vi "LinearQuadraticRegulator_New_N.vi"(4 "dt_Seconds":dbl=0.02, 5 "States":i32, 6 "N":T1, 7 "Inputs":i32, 8 "R":T1, 9 "Q":T1, 10 "B":T1, 11 "A":T1) -> (0 "Error":errorcluster, 3 "LinearQuadraticRegulator":T2)   [LabVIEW 2019, in "Trajectory_Library.lvlib"]
doc: "Contains the controller coefficients and logic for a linear-quadratic regulator (LQR). LQRs use the control law u = K(r - x).\n \nFor more on the underlying math, read https://file.tavsys.net/control/controls-engineering-in-frc.pdf.\n\nConstructs a controller with the given coefficients and plant.\n\nInputs:\n - A -- Continuous system matrix of the plant being controlled.\n - B -- Continuous input matrix of the plant being controlled.\n - Q -- The state cost matrix.\n - R -- The input cost matrix.\n - N -- The state-input cross-term cost matrix.\n - dtSeconds -- Discretization timestep.\n\nOutputs:\n - LinearQuadraticRegulator -- controller data cluster\n - Error -- if TRUE, and error occured"
uses:
  Trajectory_Library.lvlib
  <vilib>/Analysis/Matrix/Datatypes/RealMatrix.ctl
  <vilib>/Analysis/Matrix/NI_Matrix.lvlib
  TypeDef/LINEAR_QUADRATIC_REGULATOR.ctl
  <vilib>/Analysis/NI_AALPro.lvlib
  <vilib>/Analysis/NI_AALBase.lvlib
  <vilib>/Analysis/baseanly.llb/Real A x B.vi
  <vilib>/Analysis/Matrix/Numeric/Add/Add - RM,RM.vi
  <vilib>/Analysis/7linalg.llb/Real Transpose Matrix.vi
  <vilib>/Analysis/7linalg.llb/Solve Linear Equations (multiple right hand).vi
panel:
  # "<States,States>"
  # "<States,Inputs>"
  # "<States,Inputs>"
  # "<States,States>"
  # "<Inputs,Inputs>"
  # "Ref State <States,1>"
  # "Comp and capped \noutput <Inputs,1>"
  # "Controller gain\n<Inputs,States>"
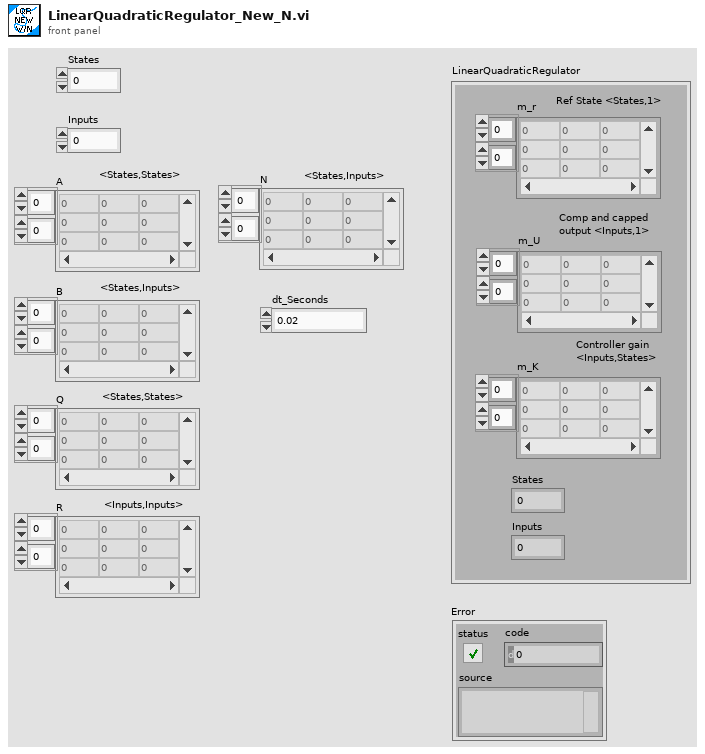
[diagram p1: front panel]
types:
  T1 = typedef "NI_Matrix.lvlib/RealMatrix.ctl" = dbl[][]
  T2 = typedef "Trajectory_Library.lvlib/LINEAR_QUADRATIC_REGULATOR.ctl" = cluster{"m_r":T1, "m_U":T1, "m_K":T1, "States":i32, "Inputs":i32}
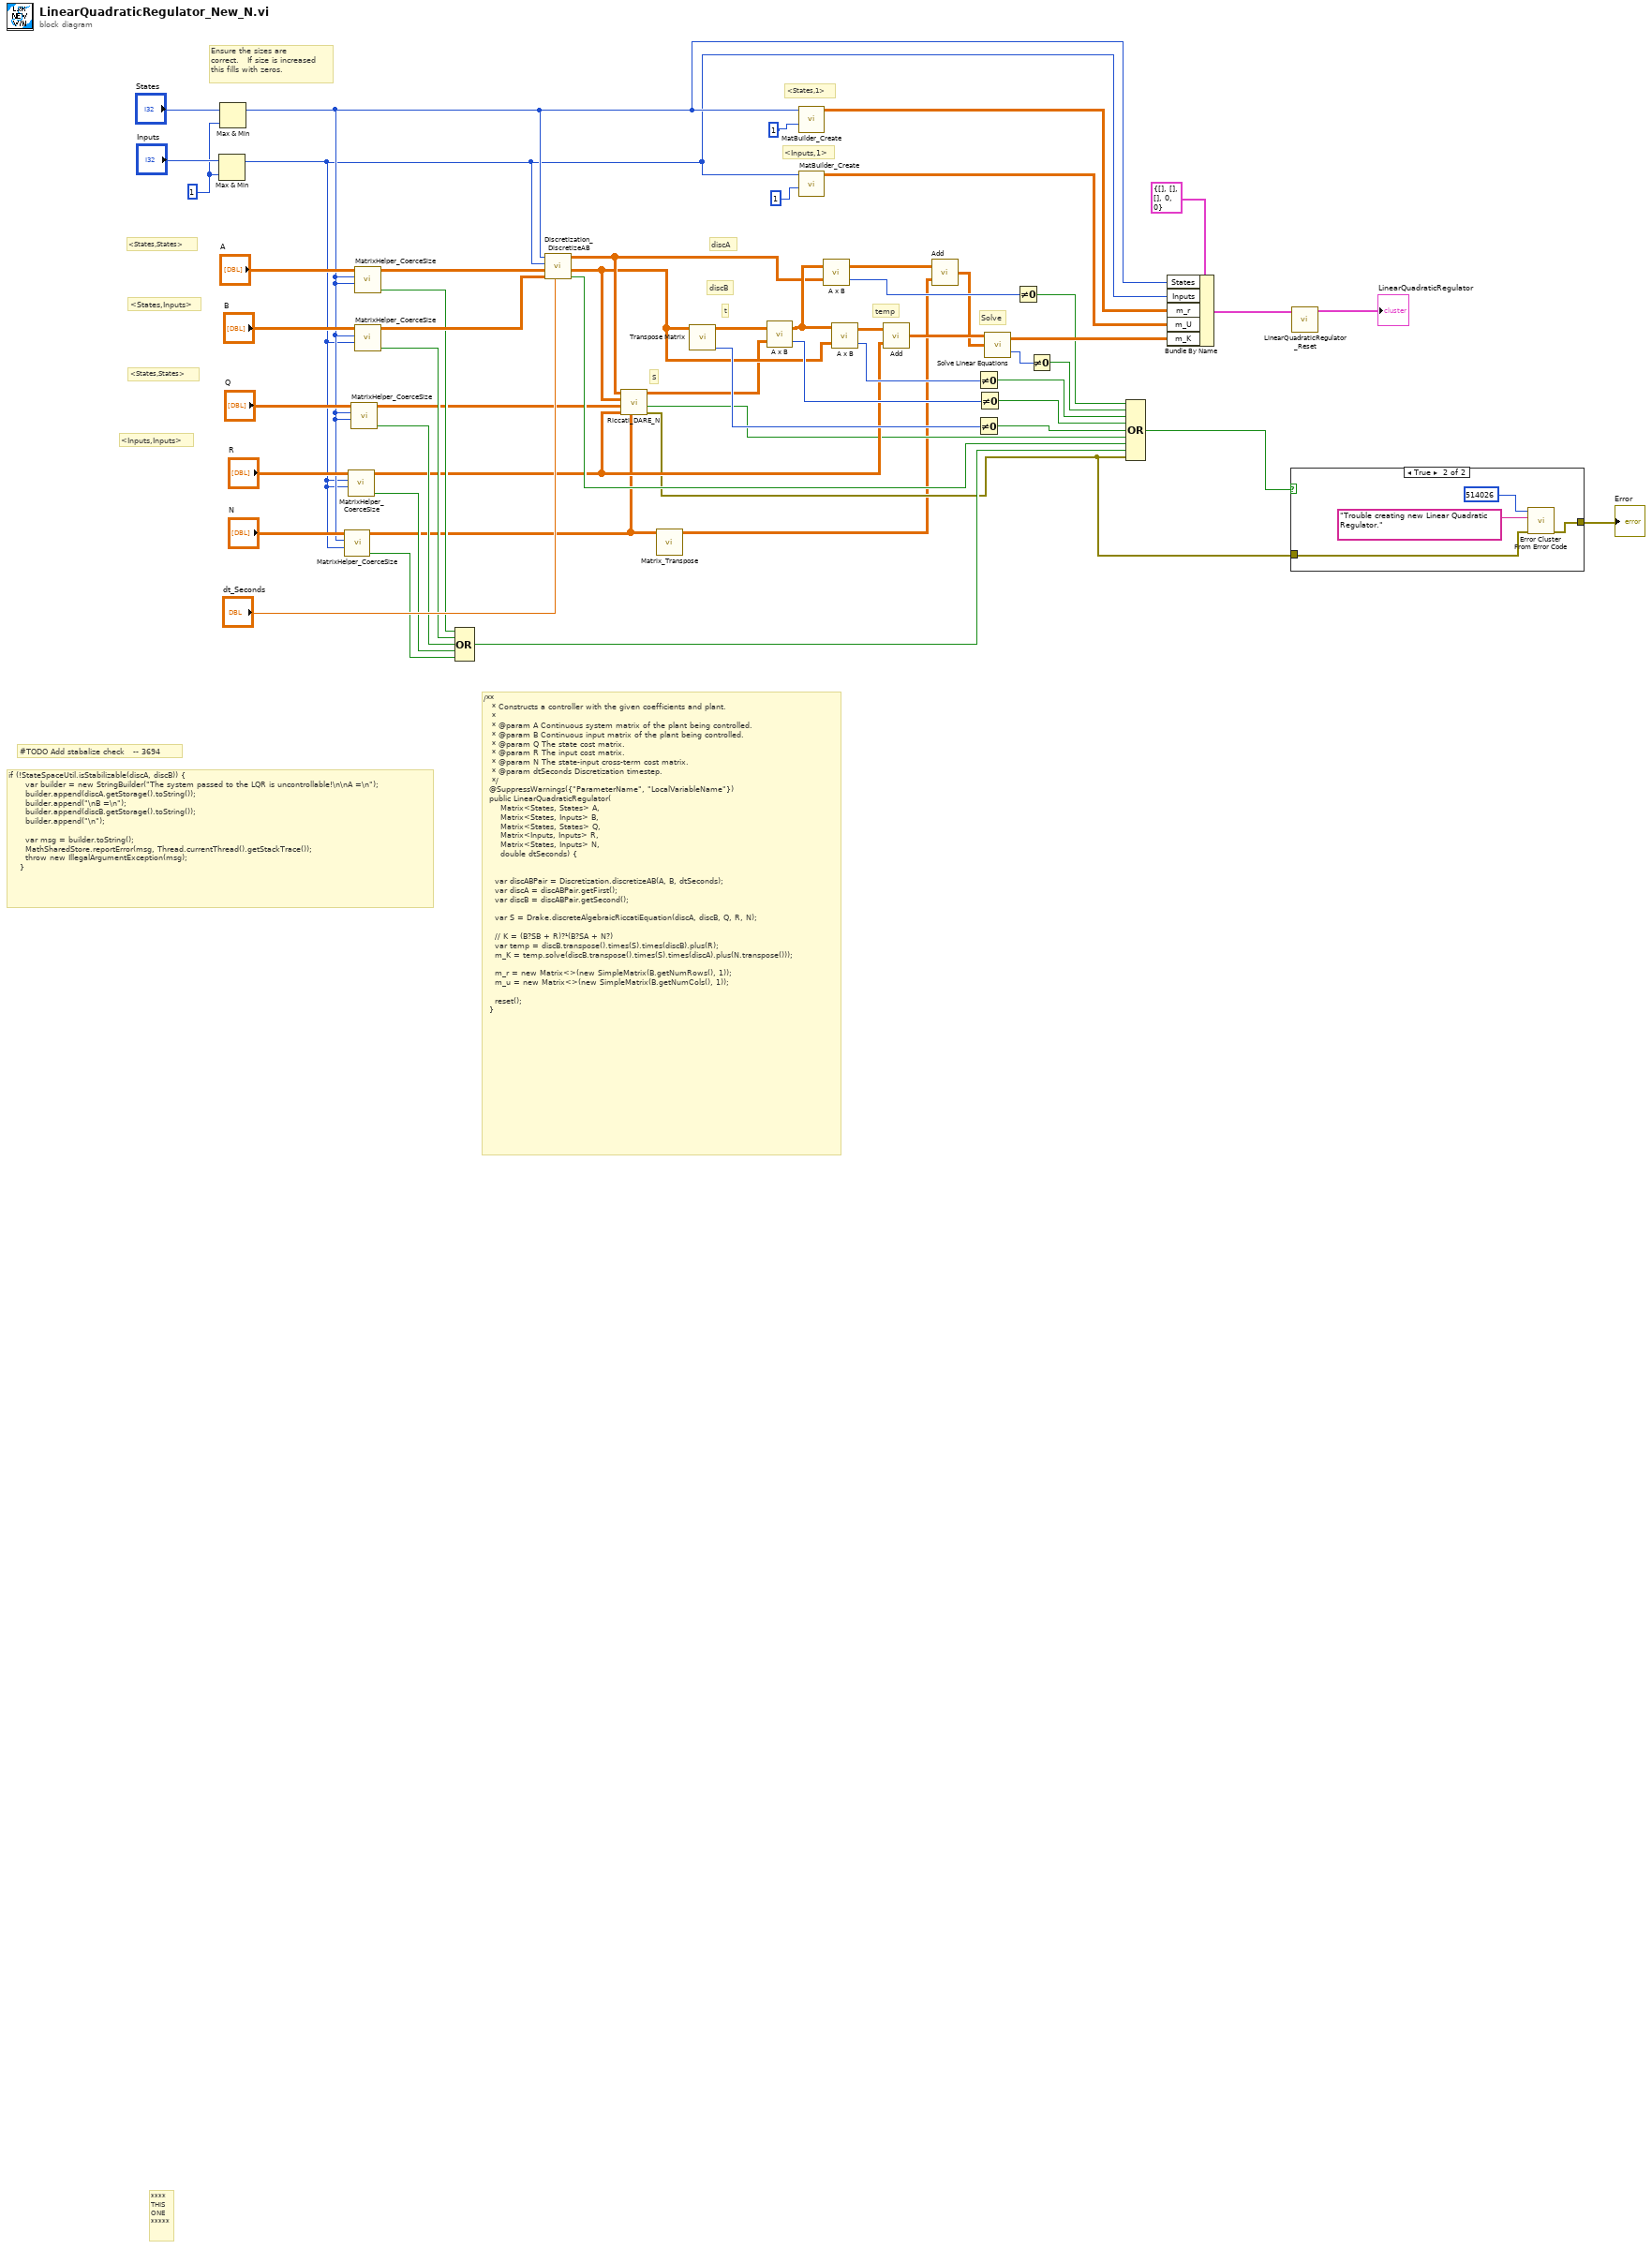
[diagram p0: block diagram]
diagram:
  w52 = 1 ("y")
  # "#TODO Add stabalize check   -- 3694"
  # "if (!StateSpaceUtil.isStabilizable(discA, discB)) {\n      var builder = new StringBuilder(\"The system passed to the LQR is uncontrollable!\\n\\nA =\\n\");\n      builder.append(discA.getStorage().toString());\n      builder.append(\"\\nB =\\n\");\n      builder.append(discB.getStorage().toString());\n      builder.append(\"\\n\");\n\n      var msg = builder.toString();\n      MathSharedStore.reportError(msg, Thread.currentThread().getStackTrace());\n      throw new IllegalArgumentException(msg);\n    }"
  # "S"
  # "Solve"
  # "t"
  # "temp"
  # "<Inputs,1>"
  # "<States,1>"
  # "discB"
  # "discA"
  # "<Inputs,Inputs>"
  # "<States,States>"
  # "<States,Inputs>"
  # "<States,States>"
  # "Ensure the sizes are\ncorrect.   If size is increased \nthis fills with zeros."
  # "/**\n   * Constructs a controller with the given coefficients and plant.\n   *\n   * @param A Continuous system matrix of the plant being controlled.\n   * @param B Continuous input matrix of the plant being controlled.\n   * @param Q The state cost matrix.\n   * @param R The input cost matrix.\n   * @param N The state-input cross-term cost matrix.\n   * @param dtSeconds Discretization timestep.\n   */\n  @SuppressWarnings({\"ParameterName\", \"LocalVariableName\"})\n  public LinearQuadraticRegulator(\n      Matrix<States, States> A,\n      Matrix<States, Inputs> B,\n      Matrix<States, States> Q,\n      Matrix<Inputs, Inputs> R,\n      Matrix<States, Inputs> N,\n      double dtSeconds) {\n\n\n    var discABPair = Discretization.discretizeAB(A, B, dtSeconds);\n    var discA = discABPair.getFirst();\n    var discB = discABPair.getSecond();\n\n    var S = Drake.discreteAlgebraicRiccatiEquation(discA, discB, Q, R, N);\n\n    // K = (B?SB + R)?¹(B?SA + N?)\n    var temp = discB.transpose().times(S).times(discB).plus(R);\n    m_K = temp.solve(discB.transpose().times(S).times(discA).plus(N.transpose()));\n\n    m_r = new Matrix<>(new SimpleMatrix(B.getNumRows(), 1));\n    m_u = new Matrix<>(new SimpleMatrix(B.getNumCols(), 1));\n\n    reset();\n  }"
  # "****\nTHIS\nONE\n*****"
  n1 = Max & Min(x="Inputs", y=w52) -> (max(x,y)=w13:i32)  [unwired: 1 out]
  n2 = Max & Min(x="States", y=w52) -> (max(x,y)=w14:i32)  [unwired: 1 out]
  n3 = call "MatrixHelper_CoerceSize.vi"("Columns"=w13, "Rows"=w14, "input matrix"="N") -> ("Coerced"=w12:bool, "output matrix"=w3:T1)  [unwired: 7 in]
  n4 = call "MatrixHelper_CoerceSize.vi"("Columns"=w13, "Rows"=w13, "input matrix"="R") -> ("Coerced"=w48:bool, "output matrix"=w7:T1)  [unwired: 7 in]
  n5 = call "MatrixHelper_CoerceSize.vi"("Columns"=w14, "Rows"=w14, "input matrix"="Q") -> ("Coerced"=w46:bool, "output matrix"=w8:T1)  [unwired: 7 in]
  n6 = call "MatrixHelper_CoerceSize.vi"("Columns"=w14, "Rows"=w14, "input matrix"="A") -> ("Coerced"=w40:bool, "output matrix"=w42:T1)  [unwired: 7 in]
  n7 = call "MatrixHelper_CoerceSize.vi"("Columns"=w13, "Rows"=w14, "input matrix"="B") -> ("Coerced"=w41:bool, "output matrix"=w44:T1)  [unwired: 7 in]
  n8 = Compound Arithmetic op=OR(w40, w41, w46, w48, w12) -> (w18:bool)
  n9 = call "Discretization_DiscretizeAB.vi"("dT_Seconds"="dt_Seconds", "ContB"=w44, "ContA"=w42, "Inputs"=w13, "States"=w14) -> ("Error"=w23:bool, "DiscB"=w9:T1, "DiscA"=w10:T1)  [unwired: 4 in]
  n10 = call "Riccati_DARE_N.vi"("N"=w3, "R"=w7, "Q"=w8, "B"=w9, "A"=w10) -> ("error out"=w4:errorcluster, "Error"=w5:bool, "Answer"=w6:T1)  [unwired: 3 in, 1 out]
  n11 = call "Matrix_Transpose.vi"("input matrix"=w3) -> ("output matrix"=w1:T1)  [unwired: 10 in]
  n12 = call-poly <vilib>:"Transpose Matrix.vi"("Input Matrix"=w9) -> ("error"=w25:i32, "Matrix Transpose"=w38:T1)  [unwired: 9 in]
  n13 = call-poly <vilib>:"A x B.vi"("B"=w6, "A"=w38) -> ("error"=w27:i32, "A x B"=w36:T1)
  n14 = call "MatBuilder_Create.vi"("Columns"=1 ("number of columns"), "Rows"=w14) -> ("output matrix"=w21:T1)  [unwired: 9 in]
  n15 = call "MatBuilder_Create.vi"("Columns"=1 ("number of columns"), "Rows"=w13) -> ("output matrix"=w20:T1)  [unwired: 9 in]
  n16 = call-poly <vilib>:"A x B.vi"("B"=w10, "A"=w36) -> ("error"=w33:i32, "A x B"=w11:T1)
  n17 = call-poly <vilib>:"A x B.vi"("B"=w9, "A"=w36) -> ("error"=w32:i32, "A x B"=w35:T1)
  n18 = call-poly <vilib>:"Add.vi"("Real Matrix B"=w7, "Real Matrix A"=w35) -> ("A + B"=w34:T1)
  n19 = call-poly <vilib>:"Add.vi"("Real Matrix B"=w1, "Real Matrix A"=w11) -> ("A + B"=w2:T1)
  n20 = Not Equal To 0?(x=w32) -> (x != 0?=w28:bool)
  n21 = Not Equal To 0?(x=w25) -> (x != 0?=w24:bool)
  n22 = Not Equal To 0?(x=w27) -> (x != 0?=w26:bool)
  n23 = call-poly <vilib>:"Solve Linear Equations.vi"("Known Matrix"=w2, "Input Matrix"=w34) -> ("error"=w31:i32, "Solution Matrix"=w37:T1)  [unwired: 1 in]
  n24 = Not Equal To 0?(x=w33) -> (x != 0?=w30:bool)
  n25 = Not Equal To 0?(x=w31) -> (x != 0?=w29:bool)
  n26 = Compound Arithmetic op=OR(w30, w29, w28, w26, w24, w5, w23, w18, w4) -> (w17:bool)
  n27 = Bundle By Name(cluster=T2 {"m_r"=[], "m_U"=[], "m_K"=[], "States"=0, "Inputs"=0} ("LINEARQUADRATICREGULATOR"), "States"=w14, "Inputs"=w13, "m_r"=w21, "m_U"=w20, "m_K"=w37) -> (w51:T2)
  n28 = case shown="True" w17 {
    tunnel: w4 -> [w56 w59]
    tunnel: [w56 w60] -> w16
    frame False {
    }
    frame True {
      n29 = call <vilib>:"Error Cluster From Error Code.vi"("error in (no error)"=w59, "error message (\"\")"="Trouble creating new Linear Quadratic Regulator." ("error message (\"\")"), "error code (0)"=514026) -> ("error out"=w60:errorcluster)  [unwired: 6 in]
    }
  }
  "Error" <- w16
  n30 = call "LinearQuadraticRegulator_Reset.vi"("in LinearQuadraticRegulator"=w51) -> ("out LinearQuadraticRegulator"=→"LinearQuadraticRegulator":T2)  [unwired: 10 in]
